vi "FailureDescription.vi"(8 "error in (no error)":errorcluster, 10 "Actual":variant, 11 "UnaryOperator in":refnum<class "UnaryOperator.lvclass">) -> (0 "error out":errorcluster, 2 "Failure Description":string, 3 "UnaryOperator out":refnum<class "UnaryOperator.lvclass">)   [LabVIEW 2017, in "Transparent Assertions.lvlib" / "Constraints.lvlib" / "UnaryOperator.lvclass"]
doc: "Return the second part of the scentence \"Failed asserting that ...\""
uses:
  UnaryOperator.lvclass
  UnaryOperator.lvclass/UnaryOperator.ctl
  Constraint/Constraint.lvclass
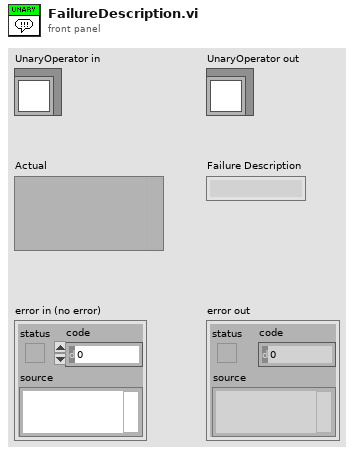
[diagram p1: front panel]
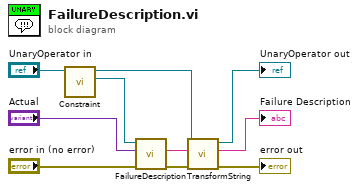
[diagram p0: block diagram]
diagram:
  n1 = call "Constraint.vi"("UnaryOperator in"="UnaryOperator in") -> ("Constraint.lvlib:Constraint.lvclass"=w1:refnum<class "Constraint.lvclass">, "UnaryOperator out"=w2:refnum<class "UnaryOperator.lvclass">)  [unwired: 9 in]
  n2 = call-dynamic "FailureDescription.vi"("error in (no error)"="error in (no error)", "Actual"="Actual", "Constraint in"=w1) -> ("error out"=w8:errorcluster, "Failure Description"=w5:string)  [unwired: 6 in, 1 out]
  n3 = call-dynamic "TransformString.vi"("error in (no error)"=w8, "String"=w5, "UnaryOperator in"=w2) -> ("error out"=→"error out":errorcluster, "String out"=→"Failure Description":string, "UnaryOperator out"=→"UnaryOperator out":refnum<class "UnaryOperator.lvclass">)  [unwired: 6 in]
